vi "BRig_dataTrial_L_Rew_event_I_l2.vi"() -> (2 "output_L_Rew_event_I_l2":i32)   [LabVIEW 2014]
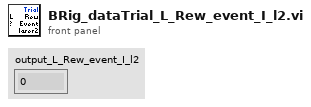
[diagram p1: front panel]
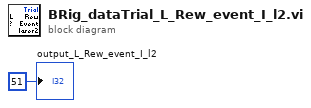
[diagram p0: block diagram]
diagram:
  "output_L_Rew_event_I_l2" <- 51 ("output_iBlock")
